vi "Test Conversion.vi"(8 "error in (no error)":errorcluster) -> (0 "error out":errorcluster)   [LabVIEW 2020]
uses:
  019fd4e5-4c5a-4d58-aa36-4c214ec7eb9c.vi
  d4f1c64c-adec-4b99-b1c3-0ed360a4b84b.vi
  9cb7cdb2-9c4b-4cf3-9f75-ac14b5b2fdc5.vi
  efb7deed-8e3f-470a-b9e5-778310688f78.vi
  9cb7cdb2-9c4b-4cf3-9f75-ac14b5b2fdc5.vi/c14c6a6c-f953-4324-9288-05fdd70fdbdd.vi
  <vilib>/Utility/error.llb/Error Cluster From Error Code.vi
  <vilib>/addons/_JKI Toolkits/Caraya/classes/Assert/Assert Equal Value_Variant.vi
  <vilib>/addons/_JKI Toolkits/Caraya/classes/Assert/Assert Equal Value and Type_Variant.vi
  <vilib>/addons/_JKI Toolkits/Caraya/classes/Test/Test.lvclass
  <vilib>/addons/_JKI Toolkits/Caraya/classes/Assert/Assert.lvclass
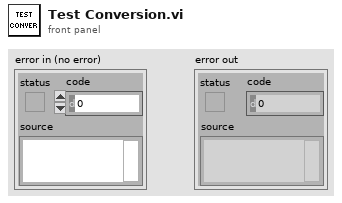
[diagram p1: front panel]
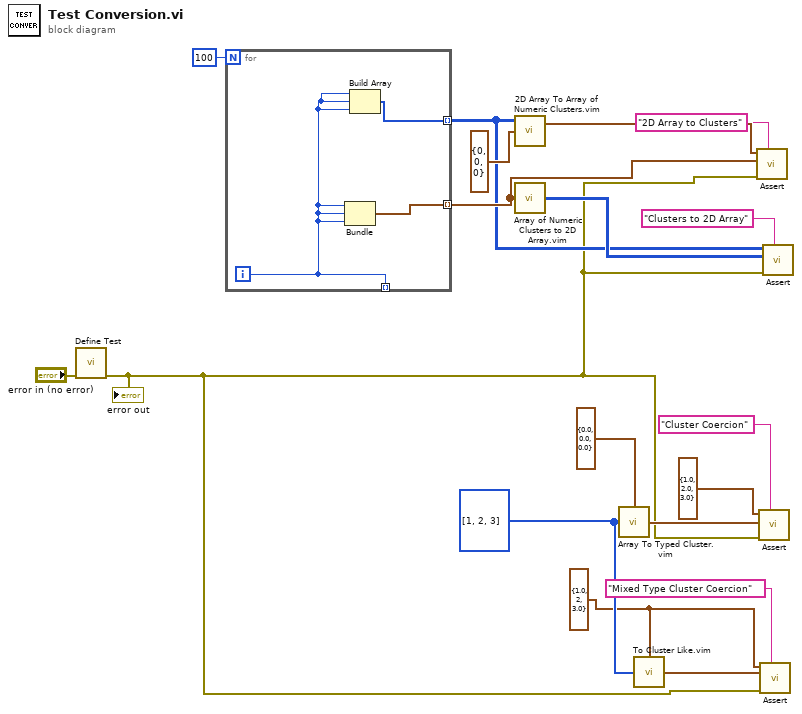
[diagram p0: block diagram]
diagram:
  w4 = cluster{dbl, i8, sgl} {1.0, 2, 3.0}
  w6 = i32[] [1, 2, 3]
  n1 = call <vilib>:"Define Test.vi"("error in (no error)"="error in (no error)") -> ("error out"=w3:errorcluster)  [unwired: 10 in]
  "error out" <- w3
  n2 = for {
    N: 100 -> [_]
    tunnel: [w21] -> w15 mode=indexing
    tunnel: [w20] -> w12 mode=indexing
    tunnel: [w19] -> _ mode=indexing
    i -> [w19]
    n3 = Bundle(w19, w19, w19) -> (w21:cluster{i32, i32, i32})  [unwired: 1 in]
    n4 = Build Array(w19, w19, w19) -> (w20:i32[])
  }
  n5 = call "2D Array To Array of Numeric Clusters.vim"("Cluster type (Rows)"=cluster{i32, i32, i32} {0, 0, 0}, "2D Array In"=w12) -> ("Array of Clusters Out"=w16:cluster{i32, i32, i32}[])  [unwired: 1 in, 1 out]
  n6 = call "Array of Numeric Clusters to 2D Array.vim"("Array of Clusters in"=w15) -> ("2D Array Out"=w14:i32[][])
  n7 = call "Array To Typed Cluster.vim"("Array"=w6, "Cluster Type"=cluster{dbl, dbl, dbl} {0.0, 0.0, 0.0}) -> ("Cluster Out"=w9:cluster{dbl, dbl, dbl})
  n8 = call "To Cluster Like.vim"("Array"=w6, "Cluster Template"=w4) -> ("Coerced Array Out"=w5:cluster{dbl, i8, sgl})
  n9 = call-poly <vilib>:"Assert.vi"("Label"="2D Array to Clusters", "error in (no error)"=w3, "Y"=w15, "X"=w16) -> ()  [unwired: 7 in, 1 out]
  n10 = call-poly <vilib>:"Assert.vi"("Label"="Cluster Coercion", "error in (no error)"=w3, "Y"=w9, "X"=cluster{dbl, dbl, dbl} {1.0, 2.0, 3.0}) -> ()  [unwired: 7 in, 1 out]
  n11 = call-poly <vilib>:"Assert.vi"("Label"="Mixed Type Cluster Coercion", "error in (no error)"=w3, "Y"=w5, "X"=w4) -> ()  [unwired: 7 in, 1 out]
  n12 = call-poly <vilib>:"Assert.vi"("Label"="Clusters to 2D Array", "error in (no error)"=w3, "Y"=w14, "X"=w12) -> ()  [unwired: 7 in, 1 out]
